vi "python.vi"() -> ()   [LabVIEW 2018]
panel:
  out "result":string
  out "에러 출력":errorcluster
  in  "함수 이름":string
  in  "모듈 경로":path
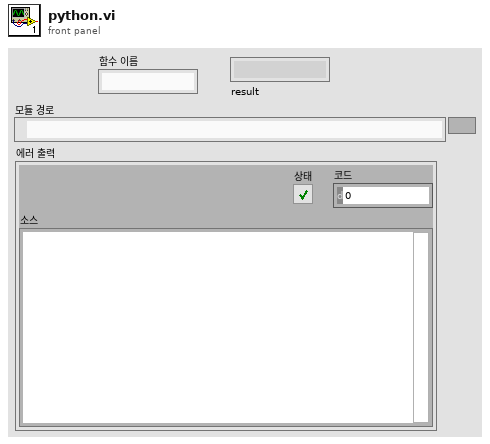
[diagram p1: front panel]
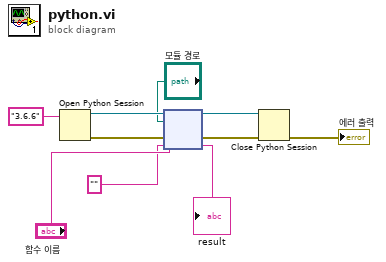
[diagram p0: block diagram]
diagram:
  n1 = Open Python Session(python version="3.6.6" ("Python 버전")) -> (session out=w7:refnum<k35>, error out=w9:errorcluster)  [unwired: 2 in]
  n2 = node(w7, "모듈 경로", "함수 이름", w9, "") -> (w4:refnum<k35>, w8:errorcluster, →"result":string)  [unwired: 2 out]
  n3 = Close Python Session(session in=w4, error in=w8) -> (11:→"에러 출력":errorcluster)
